vi "Set Power Supply.vi"(2 "Values":string, 3 "GPIB":u8, 4 "channel (ch1:0)":u16(ring) items=["channel 1", "channel 2", "channel 3"], 5 "Supply #1 Address":u8) -> (0 "error out":errorcluster, 1 "Control Voltage Status":string)   [LabVIEW 2023]
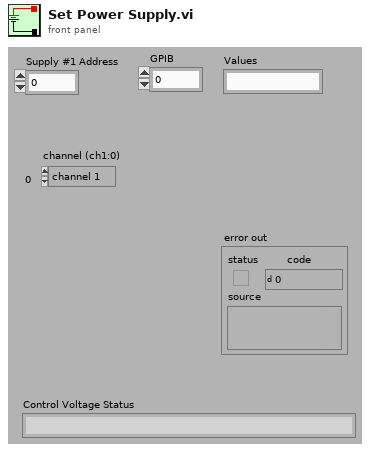
[diagram p1: front panel]
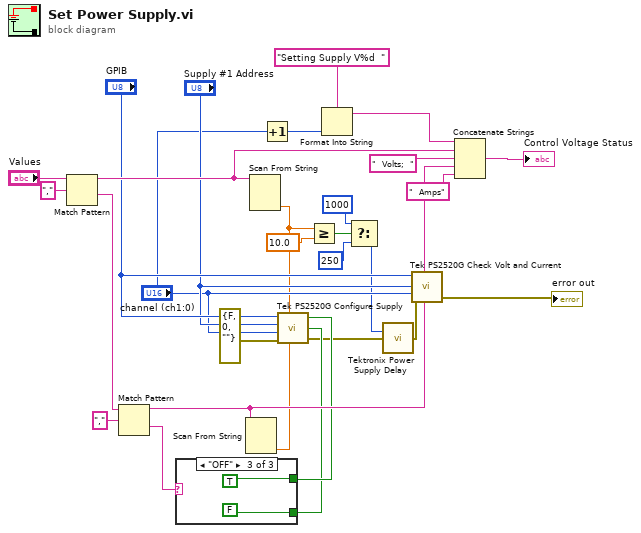
[diagram p0: block diagram]
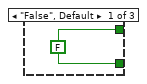
[diagram p2: hidden frame]
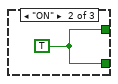
[diagram p3: hidden frame]
diagram:
  n1 = Match Pattern(string="Values", regular expression=",") -> (before substring=w21:string, after substring=w25:string)  [unwired: 1 in, 2 out]
  n2 = Match Pattern(string=w25, regular expression=",") -> (before substring=w26:string, after substring=w27:string)  [unwired: 1 in, 2 out]
  n3 = case shown="\"OFF\"" w27 {
    tunnel: [w30 w31 FALSE] -> w14
    tunnel: [w30 w31 TRUE] -> w15
    frame "False", Default {
      w30 = FALSE
    }
    frame "ON" {
      w31 = TRUE
    }
    frame "OFF" {
    }
  }
  n4 = Scan From String(input string=w26) -> (output 1=w9:dbl)  [unwired: 4 in, 3 out]
  n5 = Scan From String(input string=w21) -> (output 1=w7:dbl)  [unwired: 4 in, 3 out]
  n6 = Increment(x="channel (ch1:0)") -> (x+1=w18:u16)
  n7 = call "Tek PS2520G Configure Supply.vi"("GPIB #"="GPIB", "voltage limit"=w7, "Address"="Supply #1 Address", "channel (ch1:0)"="channel (ch1:0)", "current limit"=w9, "error in (no error)"=errorcluster {"status"=FALSE, "code"=0, "source"=""}, "Switch Output"=w15, "output (t:on)"=w14) -> ("error out"=w5:errorcluster)
  n8 = Greater Or Equal?(x=w7, y=10.0) -> (x >= y?=w4:bool)
  n9 = Format Into String(format string="Setting Supply V%d  ", w18) -> (resulting string=w16:string)  [unwired: 2 in, 1 out]
  n10 = Select(t=1000, s=w4, f=250) -> (s? t:f=w3:i32)
  n11 = call "Tektronix Power Supply Delay.vi"("error in (no error)"=w5, "Delay(msec)"=w3) -> ("error out"=w8:errorcluster)
  n12 = call "Tek PS2520G Check Volt and Current.vi"("GPIB #"="GPIB", "Address"="Supply #1 Address", "channel (ch1:0)"="channel (ch1:0)", "error in (no error)"=w8) -> ("error out"=→"error out":errorcluster)  [unwired: 2 in, 2 out]
  n13 = Concatenate Strings(w16, w21, "  Volts;  " ("Substring"), w26, "  Amps" ("Substring")) -> (→"Control Voltage Status":string)
